vi "Generate calibration profile Image references.vi"(8 "error in (no error)":errorcluster, 10 "Buffer Image Names":string[](array[string]), 11 "File Paths":path[](array[path])) -> (0 "error out":errorcluster, 2 "Image Array refs":T1[](array[typedef]))   [LabVIEW 2020]
uses:
  <vilib>/vision/Image Controls.llb/IMAQ Image.ctl
  <vilib>/vision/NI_Vision_Development_Module.lvlib
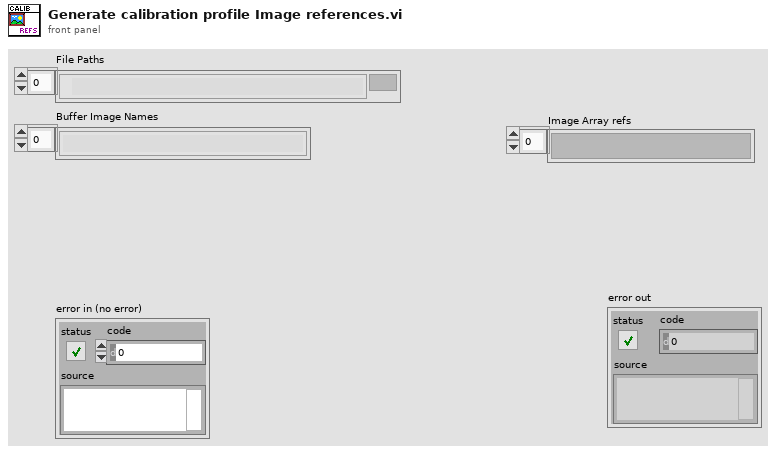
[diagram p1: front panel]
types:
  T1 = typedef "IMAQ Image.ctl" = refnum<image>
  T2 = typedef "Image Type" = u32
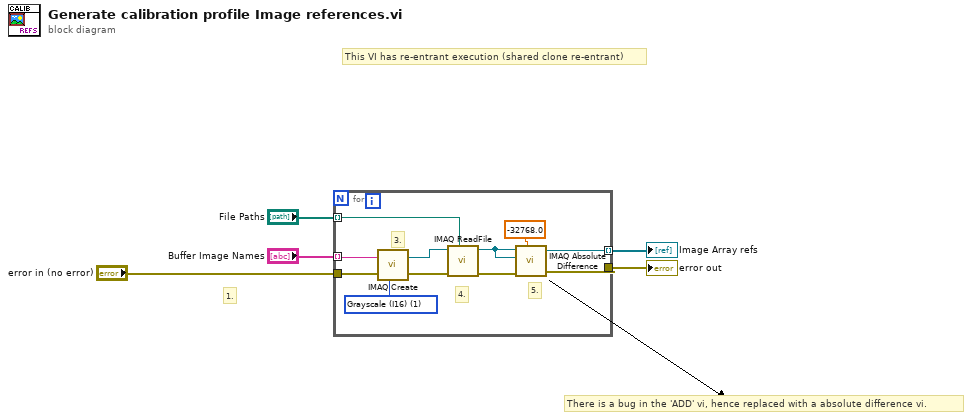
[diagram p0: block diagram]
diagram:
  # "There is a bug in the 'ADD' vi, hence replaced with a absolute difference vi."
  # "1."
  # "This VI has re-entrant execution (shared clone re-entrant)"
  n1 = for {
    tunnel: "Buffer Image Names" -> [w15] mode=indexing
    tunnel: "File Paths" -> [w11] mode=indexing
    tunnel: "error in (no error)" -> [w14]
    tunnel: [w7] -> w1 mode=indexing
    tunnel: [w6] -> w2
    w16 = T2 1 items=["Grayscale (U8)", "Grayscale (I16)", "Grayscale (SGL)", "Complex (CSG)", "RGB (U32)", "HSL (U32)", "RGB (U64)"] ("Image Type")
    # "5."
    # "4."
    # "3."
    n2 = call "IMAQ Create"("Image Name"=w15, "Image Type"=w16, "error in (no error)"=w14) -> ("New Image"=w12:T1, "error out"=w13:errorcluster)  [unwired: 2 in]
    n3 = call "IMAQ ReadFile"("File Path"=w11, "error in (no error)"=w13, "Image"=w12) -> ("error out"=w9:errorcluster, "Image Out"=w8:T1)  [unwired: 4 in, 3 out]
    n4 = call "IMAQ Absolute Difference"("Image Src A"=w8, "Constant"=-32768.0, "Image Dst"=w8, "error in (no error)"=w9) -> ("Image Dst Out"=w7:T1, "error out"=w6:errorcluster)  [unwired: 3 in]
  }
  "error out" <- w2
  "Image Array refs" <- w1
